vi "Vi 1.vi"() -> ()   [LabVIEW 2010]
panel:
  in  "stop":bool
  out "Thermometer":dbl(slide) scale=0.0..100.0
  out "Meter":dbl(knob) scale=0.0..10.0
  out "Tank":dbl(slide) scale=0.0..100.0
  in  "Numeric 2":i16
  in  "Numeric":i16
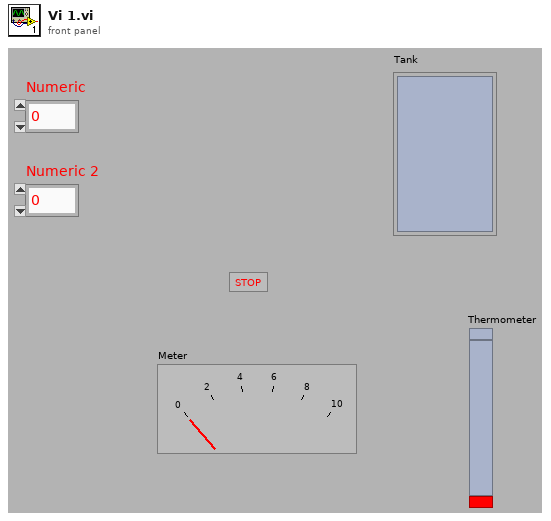
[diagram p1: front panel]
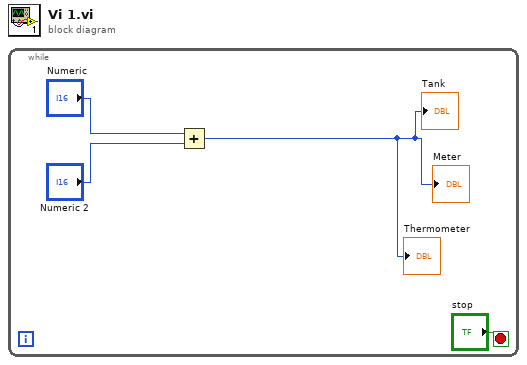
[diagram p0: block diagram]
diagram:
  n1 = while {
    stop <- "stop" stop-if-true
    n2 = Add(x="Numeric", y="Numeric 2") -> (x+y=→"Tank" →"Meter" →"Thermometer":i16)
  }
